vi "Build Tree.vi"(8 "error in (no error)":errorcluster, 10 "Tree Reference":refnum<vi>, 11 "Base Tree in":refnum<class "Base Tree.lvclass">) -> (0 "error out":errorcluster, 3 "Base Tree out":refnum<class "Base Tree.lvclass">)   [LabVIEW 2017, in "Browser Core.lvlib" / "Base Tree.lvclass"]
doc: "Write Tree hierarchy to input control reference. The Tree's root node will be used as the top level item."
uses:
  Base Tree.lvclass
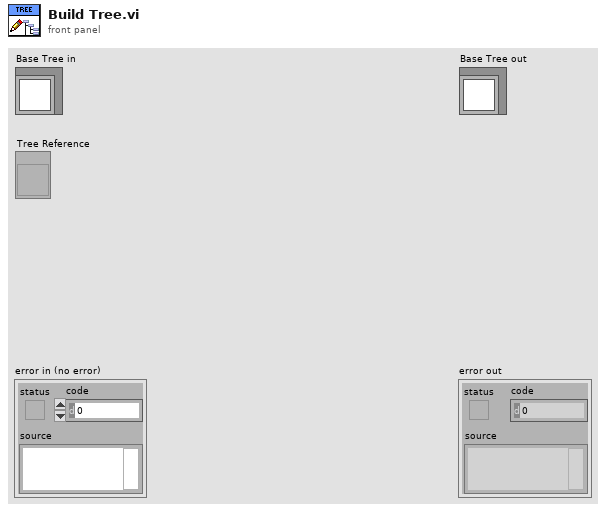
[diagram p1: front panel]
types:
  T1 = cluster{"Left Cell String":string, "Child Text":string[], "Child Tag":string, "Item Indent":i32, "Child Only?":bool, "Glyph Index":i32}[]
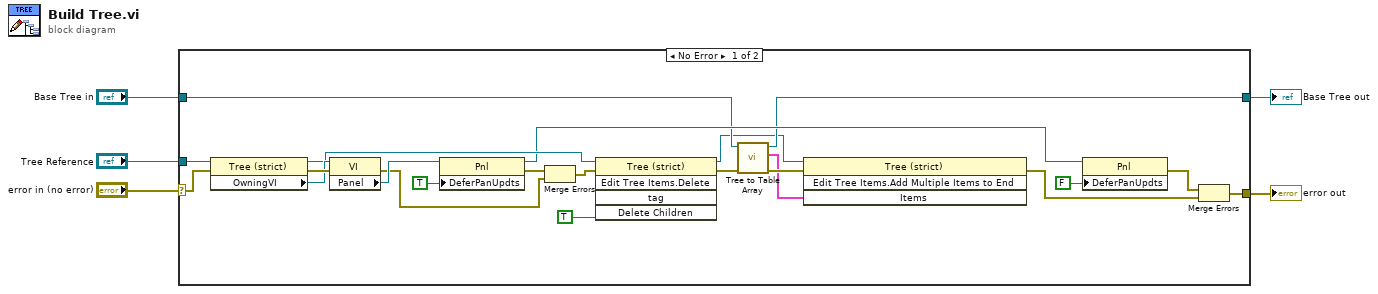
[diagram p0: block diagram]
diagram:
  n1 = case shown="No Error" "error in (no error)" {
    selector: "error in (no error)" -> [w15 w29]
    tunnel: [w13 w29] -> w4
    tunnel: [w8 w28] -> w2
    tunnel: "Base Tree in" -> [w9 w28]
    tunnel: "Tree Reference" -> [w20 _]
    frame No Error {
      n2 = property class="Tree (strict)"(reference=w20, error in=w15) -> (reference out=w19:refnum<vi>, error out=w27:errorcluster, "OwningVI"=w26:refnum<vi>)
      n3 = property class="VI"(reference=w26, error in=w27) -> (error out=w16:errorcluster, "Panel"=w23:refnum<vi>)  [unwired: 1 out]
      n4 = property class="Pnl"(reference=w23, "DeferPanUpdts"=TRUE ("Defer Panel Updates")) -> (reference out=w18:refnum<vi>, error out=w22:errorcluster)  [unwired: 1 in]
      n5 = Merge Errors(w22, w16) -> (w17:errorcluster)
      n6 = invoke class="Tree (strict)" method="Edit Tree Items.Delete"(reference=w19, error in=w17, "Delete Children"=TRUE ("Delete Children?")) -> (reference out=w6:refnum<vi>, error out=w11:errorcluster)  [unwired: 2 in, 3 out]
      n7 = call-dynamic "Tree to Table Array.vi"("error in (no error)"=w11, "Base Tree in"=w9) -> ("error out"=w10:errorcluster, "Items"=w7:T1, "Base Tree out"=w8:refnum<class "Base Tree.lvclass">)  [unwired: 7 in]
      n8 = invoke class="Tree (strict)" method="Edit Tree Items.Add Multiple Items to End"(reference=w6, error in=w10, "Items"=w7) -> (error out=w12:errorcluster)  [unwired: 1 in, 3 out]
      n9 = property class="Pnl"(reference=w18, "DeferPanUpdts"=FALSE ("Defer Panel Updates")) -> (error out=w14:errorcluster)  [unwired: 1 in, 1 out]
      n10 = Merge Errors(w14, w12) -> (w13:errorcluster)
    }
    frame Error {
      # "Do Not Edit Tree on Error In"
    }
  }
  "error out" <- w4
  "Base Tree out" <- w2
